vi "beginPreparePassInGame1.vi"(6 "AnyPlayChosen?":bool, 8 "error in (no error)":errorcluster, 10 "Game in 2":refnum<class "Game.lvclass">, 11 "PreparePassInGame1 in":refnum<class "PreparePassInGame1.lvclass">) -> (0 "error out":errorcluster, 1 "begin?":bool, 3 "PreparePassInGame1 out":refnum<class "PreparePassInGame1.lvclass">)   [LabVIEW 2020, in "PreparePassInGame1.lvclass"]
uses:
  PreparePassInGame1.lvclass
  Game_class/Game.lvclass
  Team_class/OffensivePlay.ctl
  Game_class/Game.lvclass/Game.ctl
  Team_class/Team.lvclass/Team.ctl
  Game_class/Read OffensiveTeam.vi
  Team_class/Read OffensivePlay.vi
  Ally_class/Ally.lvclass
  C:/Users/Administrator/Desktop/SSL/SSL_AI/Team_class/Team.lvclass
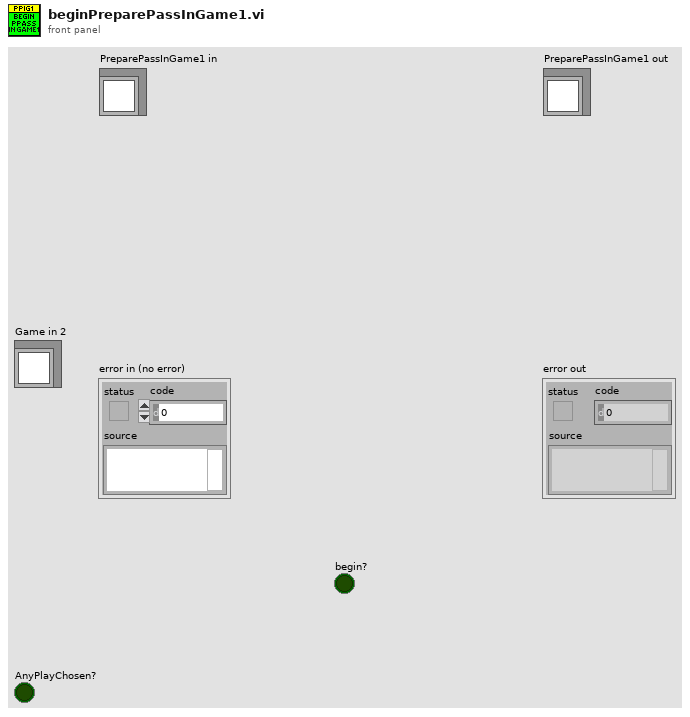
[diagram p1: front panel]
types:
  T1 = typedef "OffensivePlay.ctl" = enum16{"PrepareFourthPass", "KeeperPassToStriker", "PrepareKeeperPass", "ACBPass", "ABCPass", "PrepareTriplePass", "TableWithStriker", "TableWith2ndStrikerPlay", "PrepareDoublePass", "PrepareRollToPass", "SimplePass", "PreparePass", "PassToStriker", "BallOutOfField", "PassTo2ndStriker", "StopOffensive", "Prepare Penalty Enemy", "EnemyPossessionAtEnemyField", "EnemyPossesionAtOurField", "TestPlay", "PreparePenaltyAlly", "KickPenaltyAlly", "PrepareKickoffAlly", "PrepareKickoffEnemy", "IndirectEnemy", "DirectEnemy", "PreparePassInGame1", "NormalGame", "DirectKick", "Pass", "Halt", "Timeout", "PassPlay", "PenaltyEnemy"}
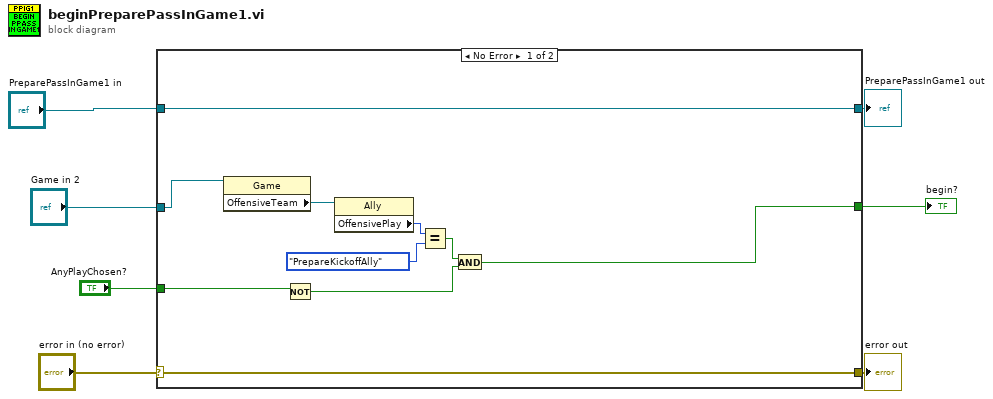
[diagram p0: block diagram]
diagram:
  n1 = case shown="No Error" "error in (no error)" {
    selector: "error in (no error)" -> [w17 w19]
    tunnel: [w17 w19] -> w6
    tunnel: [w15 w18] -> w4
    tunnel: "PreparePassInGame1 in" -> [w15 w18]
    tunnel: "AnyPlayChosen?" -> [w16 _]
    tunnel: [w8 _] -> w2
    tunnel: "Game in 2" -> [w13 _]
    frame No Error {
      n2 = property class="Game"(reference=w13) -> ("OffensiveTeam"=w12:refnum<class "Ally.lvclass">)  [unwired: 1 in, 2 out]
      n3 = Not(x=w16) -> (.not. x?=w14:bool)
      n4 = property class="Ally"(reference=w12) -> ("OffensivePlay"=w11:T1)  [unwired: 1 in, 2 out]
      n5 = Equal?(x=w11, y=OffensivePlay."PrepareKickoffAlly" ("OffensivePlay")) -> (x = y?=w9:bool)
      n6 = And(x=w9, y=w14) -> (x .and. y?=w8:bool)
    }
    frame Error {
    }
  }
  "error out" <- w6
  "PreparePassInGame1 out" <- w4
  "begin?" <- w2
